vi "serial.COM.dialog.vi"(10 "Arduino COM":refnum<visa-resource-name>="COM5") -> (1 "cancel out":bool, 2 "COM out":refnum<visa-resource-name>, 4 "quit out":bool)   [LabVIEW 2020]
panel:
  in  "cancel":bool
  in  "quit":bool
  in  "ok":bool
  # "Could not connect to Arduino\nWould you like to change COM port?"
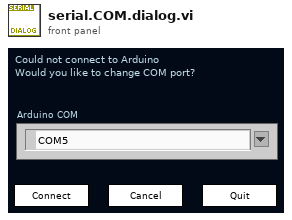
[diagram p1: front panel]
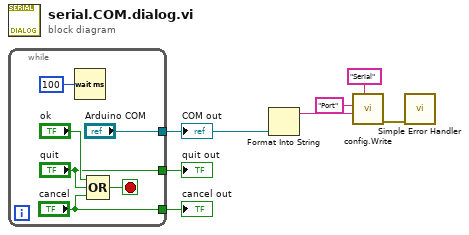
[diagram p0: block diagram]
diagram:
  n1 = while {
    tunnel: ["Arduino COM"] -> w3
    tunnel: ["quit"] -> w7
    tunnel: ["cancel"] -> w6
    stop <- w12 stop-if-true
    n2 = Wait (ms)(milliseconds to wait=u32 100) -> ()  [unwired: 1 out]
    n3 = Compound Arithmetic op=OR("ok", "quit", "cancel") -> (w12:bool)
  }
  "COM out" <- w3
  "quit out" <- w7
  "cancel out" <- w6
  n4 = Format Into String(w3) -> (resulting string=w1:string)  [unwired: 3 in, 1 out]
  n5 = call "config.Write.vi"("section"="Serial", "value"=w1, "key"="Port") -> ("error out"=w2:errorcluster)  [unwired: 8 in]
  n6 = call <vilib>:"Simple Error Handler.vi"("error in (no error)"=w2) -> ()  [unwired: 4 in, 5 out]
